vi "Module template.vi"(0 "Static input":T1(array[cluster])=[{"Times"=[], "Voltages"=[], "Enable Ch"=TRUE, "Hinge Points"=0}, {"Times"=[], "Voltages"=[], "Enable Ch"=TRUE, "Hinge Points"=0}, {"Times"=[], "Voltages"=[], "Enable Ch"=TRUE, "Hinge Points"=0}, {"Times"=[], "Voltages"=[], "Enable Ch"=TRUE, "Hinge Points"=0}, {"Times"=[], "Voltages"=[], "Enable Ch"=TRUE, "Hinge Points"=0}, {"Times"=[], "Voltages"=[], "Enable Ch"=TRUE, "Hinge Points"=0}, {"Times"=[], "Voltages"=[], "Enable Ch"=TRUE, "Hinge Points"=0}, {"Times"=[], "Voltages"=[], "Enable Ch"=TRUE, "Hinge Points"=0}, {"Times"=[], "Voltages"=[], "Enable Ch"=TRUE, "Hinge Points"=0}, {"Times"=[], "Voltages"=[], "Enable Ch"=TRUE, "Hinge Points"=0}, {"Times"=[], "Voltages"=[], "Enable Ch"=TRUE, "Hinge Points"=0}, {"Times"=[], "Voltages"=[], "Enable Ch"=TRUE, "Hinge Points"=0}, {"Times"=[], "Voltages"=[], "Enable Ch"=TRUE, "Hinge Points"=0}, {"Times"=[], "Voltages"=[], "Enable Ch"=TRUE, "Hinge Points"=0}, {"Times"=[], "Voltages"=[], "Enable Ch"=TRUE, "Hinge Points"=0}, {"Times"=[], "Voltages"=[], "Enable Ch"=TRUE, "Hinge Points"=0}, {"Times"=[], "Voltages"=[], "Enable Ch"=FALSE, "Hinge Points"=0}, {"Times"=[], "Voltages"=[], "Enable Ch"=FALSE, "Hinge Points"=0}, {"Times"=[], "Voltages"=[], "Enable Ch"=FALSE, "Hinge Points"=0}, {"Times"=[], "Voltages"=[], "Enable Ch"=FALSE, "Hinge Points"=0}, {"Times"=[], "Voltages"=[], "Enable Ch"=FALSE, "Hinge Points"=0}, {"Times"=[], "Voltages"=[], "Enable Ch"=FALSE, "Hinge Points"=0}, {"Times"=[], "Voltages"=[], "Enable Ch"=FALSE, "Hinge Points"=0}, {"Times"=[], "Voltages"=[], "Enable Ch"=TRUE, "Hinge Points"=0}] {"Voltages" format="%.2f"; "Times" format="%.2f"}, 1 "Absolute start time (ms)":dbl=1500.0 format="%.3f", 2 "GPIB Input":T3(array[cluster]) {"Module" items=["TTL high                                                                                 ", "TTL low                          ", "Camera Strobe                   ", "CMOT", "Defaults                           ", "Fluorescence pulse           ", "IP trap                         ", "Kinetics OD image          ", "Kinetics picture", "Kinetics probe pulse", "MOT light only                ", "MOT off                                   ", "MOT on                         ", "Move cart                      ", "OD image                     ", "Optical pumping          ", "Picture                             ", "Probe Pulse", "Quadrupole trap             ", "IP off", "Utility Module 02           ", "Utility Module 03           ", "Molasses          ", "Utility Module 04     ", "Utility Module 05     ", "Utility Module 06     ", "Utility Module 07     ", "Utility Module 08     ", "Utility Module 09     ", "Utility Module 10     ", "Static DAC", "GPIB"]; "Abs Start Time" format="%.3f"}, 3 "Read/Write":bool, 5 "Input":i64[][](array[numeric]), 7 "Static DAC Linear Ramps":T5(array[cluster]) {"DAC Channel" items=["0", "1", "2", "3", "4", "5", "6", "7", "8", "9", "10", "11", "12", "13", "14", "15", "16", "17", "18", "19", "20", "21", "22", "23"]}, 9 "Manual Array":T6(array[cluster])=[{"Time2 (ms)"="100", "Port2"=4, "Line2"=23, "Comments2"="", "Value2"=FALSE, "Enable2"=TRUE, "DAC value"="1"}, {"Time2 (ms)"="200", "Port2"=4, "Line2"=23, "Comments2"="", "Value2"=FALSE, "Enable2"=TRUE, "DAC value"="2"}] {"Line2" items=["0", "1", "2", "3", "4", "5", "6", "7", "8", "9", "10", "11", "12", "13", "14", "15", "16", "17", "18", "19", "20", "21", "22", "23", "24", "25", "26", "27", "28", "29", "30", "31"]; "Port2" items=["A", "B", "C", "D", "DAC", "GPIB"]}, 10 "Do Write/Read":bool, 12 "Do this?":bool=TRUE, 14 "filename":string="Utility Module 1") -> (4 "Static output":T1(array[cluster])=[{"Times"=[], "Voltages"=[], "Enable Ch"=TRUE, "Hinge Points"=0}, {"Times"=[], "Voltages"=[], "Enable Ch"=TRUE, "Hinge Points"=0}, {"Times"=[], "Voltages"=[], "Enable Ch"=TRUE, "Hinge Points"=0}, {"Times"=[], "Voltages"=[], "Enable Ch"=TRUE, "Hinge Points"=0}, {"Times"=[], "Voltages"=[], "Enable Ch"=TRUE, "Hinge Points"=0}, {"Times"=[], "Voltages"=[], "Enable Ch"=TRUE, "Hinge Points"=0}, {"Times"=[], "Voltages"=[], "Enable Ch"=TRUE, "Hinge Points"=0}, {"Times"=[], "Voltages"=[], "Enable Ch"=TRUE, "Hinge Points"=0}, {"Times"=[], "Voltages"=[], "Enable Ch"=TRUE, "Hinge Points"=0}, {"Times"=[], "Voltages"=[], "Enable Ch"=TRUE, "Hinge Points"=0}, {"Times"=[], "Voltages"=[], "Enable Ch"=TRUE, "Hinge Points"=0}, {"Times"=[], "Voltages"=[], "Enable Ch"=TRUE, "Hinge Points"=0}, {"Times"=[], "Voltages"=[], "Enable Ch"=TRUE, "Hinge Points"=0}, {"Times"=[], "Voltages"=[], "Enable Ch"=TRUE, "Hinge Points"=0}, {"Times"=[], "Voltages"=[], "Enable Ch"=TRUE, "Hinge Points"=0}, {"Times"=[], "Voltages"=[], "Enable Ch"=TRUE, "Hinge Points"=0}] {"Voltages" format="%.2f"; "Times" format="%.2f"}, 6 "Output":i64[][](array[numeric])=[[1700001, 3, 31, 0], [1700000, 3, 31, 1], [1600001, 3, 31, 0], [1600000, 3, 31, 1]], 13 "GPIB Output":T3(array[cluster]) {"Module" items=["TTL high                                                                                 ", "TTL low                          ", "Camera Strobe                   ", "CMOT", "Defaults                           ", "Fluorescence pulse           ", "IP trap                         ", "Kinetics OD image          ", "Kinetics picture", "Kinetics probe pulse", "MOT light only                ", "MOT off                                   ", "MOT on                         ", "Move cart                      ", "OD image                     ", "Optical pumping          ", "Picture                             ", "Probe Pulse", "Quadrupole trap             ", "IP off", "Utility Module 02           ", "Utility Module 03           ", "Molasses          ", "Utility Module 04     ", "Utility Module 05     ", "Utility Module 06     ", "Utility Module 07     ", "Utility Module 08     ", "Utility Module 09     ", "Utility Module 10     ", "Static DAC", "GPIB"]; "Abs Start Time" format="%.3f"}, 15 "Saved Cluster":T4={"Manual Array"=[{"Time2 (ms)"=100.0, "Port2"=4, "Line2"=23, "Comments2"="", "Value2"=FALSE, "Enable2"=TRUE, "DAC value"=1.0}, {"Time2 (ms)"=200.0, "Port2"=4, "Line2"=23, "Comments2"="", "Value2"=FALSE, "Enable2"=TRUE, "DAC value"=2.0}], "Static DAC Linear Ramps"=[]})   [LabVIEW 2017]
uses:
  globals/Modules global.vi
  globals/DIO board parameters global.vi
  globals/RIO and DAC defaults global.vi
panel:
  out "Static input 2":T1(array[cluster])
  out "Array":T2(array[cluster])=[{"Time2 (ms)"=100.0, "Port2"=4, "Line2"=23, "Comments2"="", "Value2"=FALSE, "Enable2"=TRUE, "DAC value"=1.0}, {"Time2 (ms)"=200.0, "Port2"=4, "Line2"=23, "Comments2"="", "Value2"=FALSE, "Enable2"=TRUE, "DAC value"=2.0}]
  out "Path":path=path "E:/Debbie/experiment stuff/B231/24 Experiment Control/modules and sub-vi's/quad trap"
  out "appended path":path=path "E:/Debbie/experiment stuff/B231/24 Experiment Control/modules and sub-vi's/backups/Helmholtz1 28_Apr_2006"
  out "Comments":string[](array[string])
  out "Value":bool[](array[boolean])
  out "Line":i32[](array[numeric])
  out "Port":i32[](array[numeric])
  out "Time":dbl[](array[numeric]) format="%.3f"
  # "manual button (not connected on icon)\nIf you set this to True, be sure to set it back to False afterward."
  # "Time                   Port        Line       Value  Enable  DAC voltage  Comments"
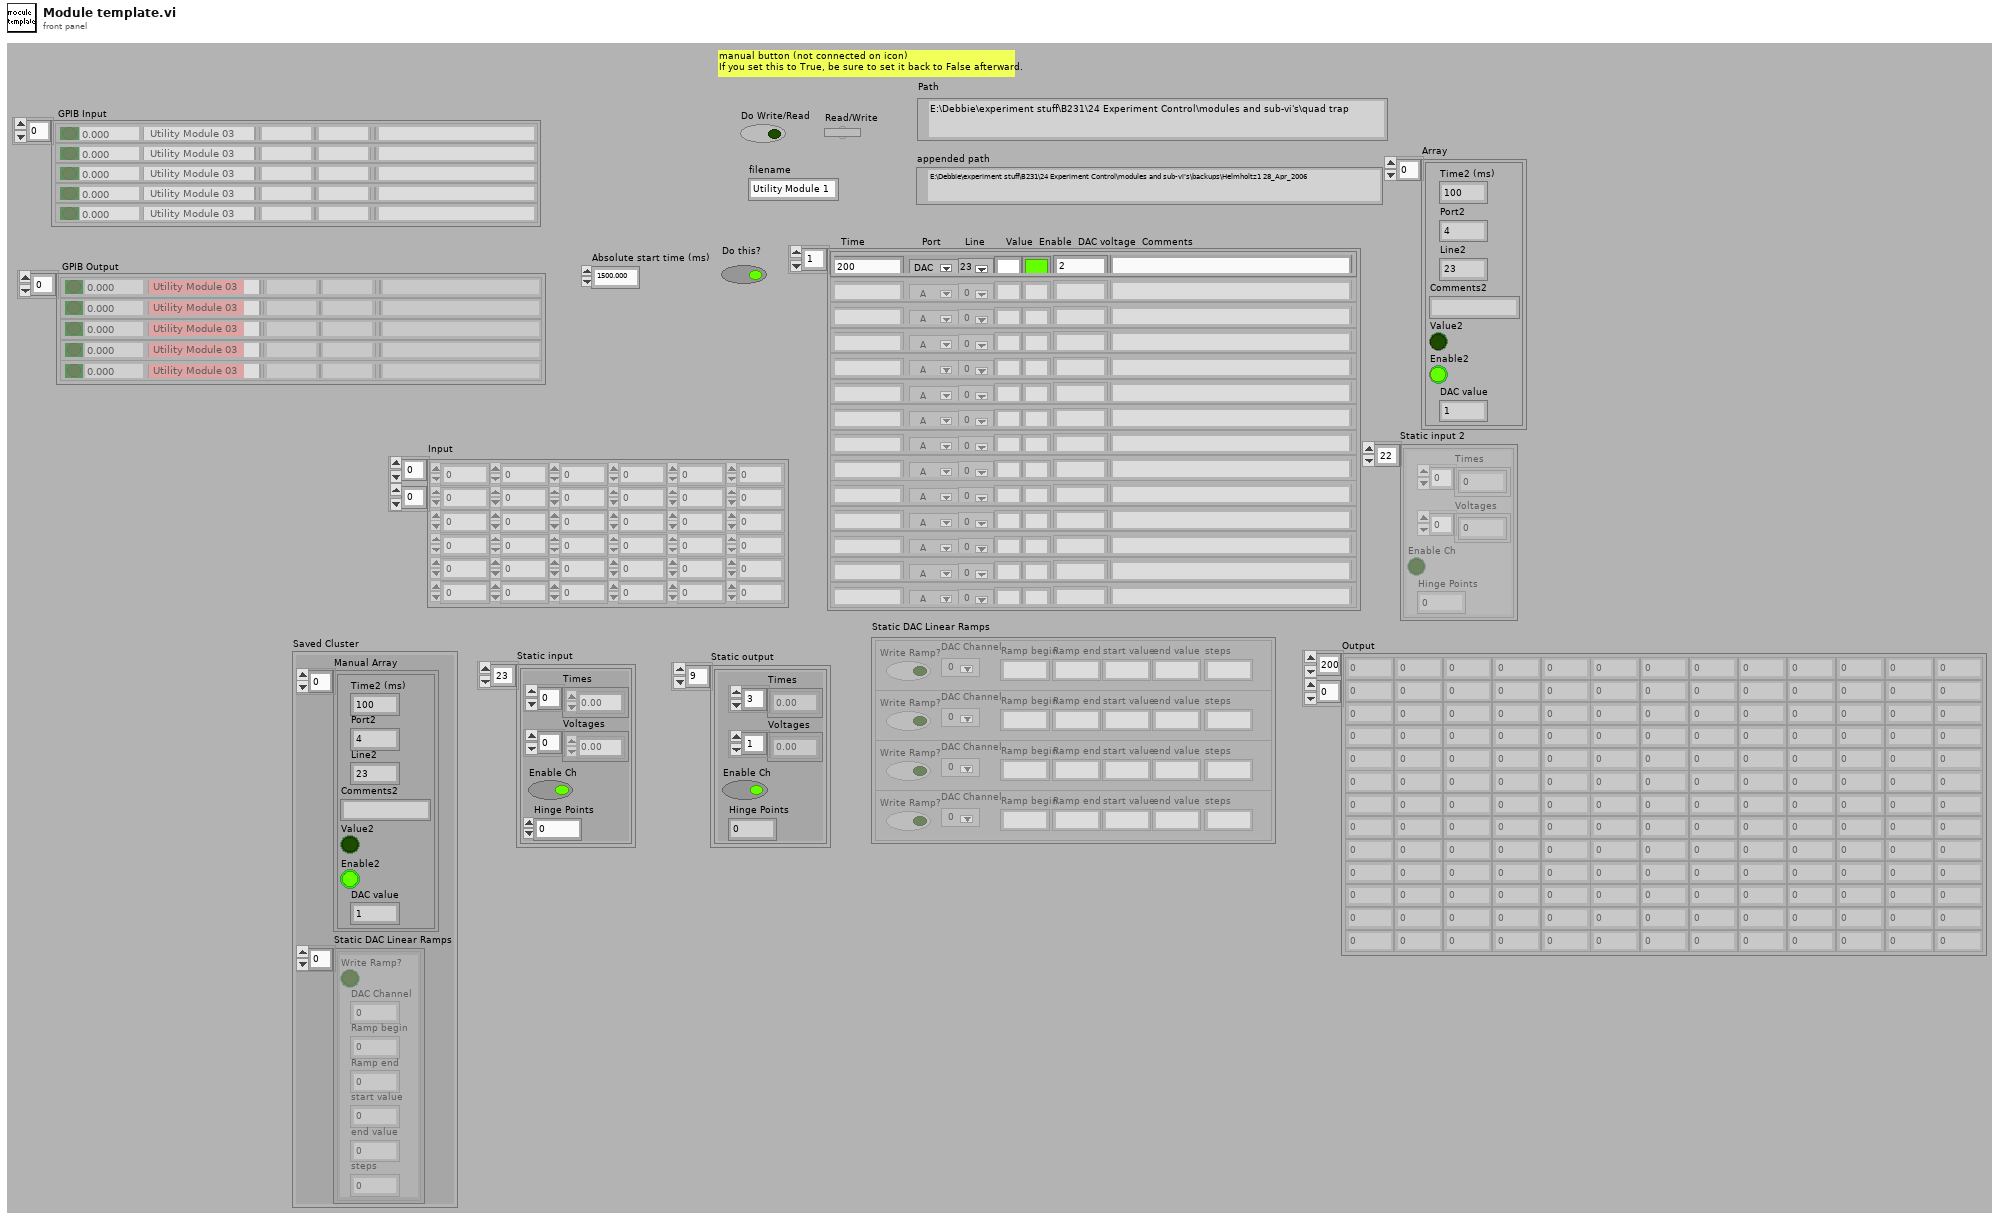
[diagram p1: front panel]
types:
  T1 = cluster{"Times":dbl[], "Voltages":dbl[], "Enable Ch":bool, "Hinge Points":u8}[]
  T2 = cluster{"Time2 (ms)":dbl, "Port2":u16, "Line2":u16, "Comments2":string, "Value2":bool, "Enable2":bool, "DAC value":dbl}[]
  T3 = cluster{"Enable":bool, "Abs Start Time":dbl, "Module":u16, "String":string, "Array":string[]}[]
  T4 = cluster{"Manual Array":cluster{"Time2 (ms)":dbl, "Port2":u16, "Line2":u16, "Comments2":string, "Value2":bool, "Enable2":bool, "DAC value":dbl}[], "Static DAC Linear Ramps":cluster{"Write Ramp?":bool, "DAC Channel":i16, "Ramp begin":dbl, "Ramp end":dbl, "start value":dbl, "end value":dbl, "steps":i16}[]}
  T5 = cluster{"Write Ramp?":bool, "DAC Channel":i16, "Ramp begin":string, "Ramp end":string, "start value":string, "end value":string, "steps":string}[]
  T6 = cluster{"Time2 (ms)":string, "Port2":u16, "Line2":u16, "Comments2":string, "Value2":bool, "Enable2":bool, "DAC value":string}[]
  T7 = cluster{"Write Ramp?":bool, "DAC Channel":i16, "Ramp begin":dbl, "Ramp end":dbl, "start value":dbl, "end value":dbl, "steps":i16}[]
  T8 = cluster{"Write Ramp?":bool, "DAC Channel":i16, "Ramp begin":dbl, "Ramp end":dbl, "start value":dbl, "end value":dbl, "steps":i16}
  T9 = cluster{"Time2 (ms)":dbl, "Port2":u16, "Line2":u16, "Comments2":string, "Value2":bool, "Enable2":bool, "DAC value":dbl}
  T10 = cluster{cluster{"Time2 (ms)":dbl, "Port2":u16, "Line2":u16, "Comments2":string, "Value2":bool, "Enable2":bool, "DAC value":dbl}[], cluster{"Write Ramp?":bool, "DAC Channel":i16, "Ramp begin":dbl, "Ramp end":dbl, "start value":dbl, "end value":dbl, "steps":i16}[]}
  T11 = enum32{"existing file", "new file", "new or existing file", "existing dir", "new dir", "new or existing dir", "existing file (use LLBs)", "new file (use LLBs)", "new or existing file (use LLBs)", "new or existing file or directory (use LLBs)"}
  T12 = enum16{"open", "replace", "create", "open or create", "replace or create", "replace or create with confirmation"}
  T13 = cluster{"Time2 (ms)":string, "Port2":u16, "Line2":u16, "Comments2":string, "Value2":bool, "Enable2":bool, "DAC value":string}
  T14 = cluster{"Write Ramp?":bool, "DAC Channel":i16, "Ramp begin":string, "Ramp end":string, "start value":string, "end value":string, "steps":string}
  T15 = cluster{"Enable":bool, "Abs Start Time":dbl, "Module":u16, "String":string, "Array":string[]}
  T16 = cluster{"Times":dbl[], "Voltages":dbl[], "Enable Ch":bool, "Hinge Points":u8}
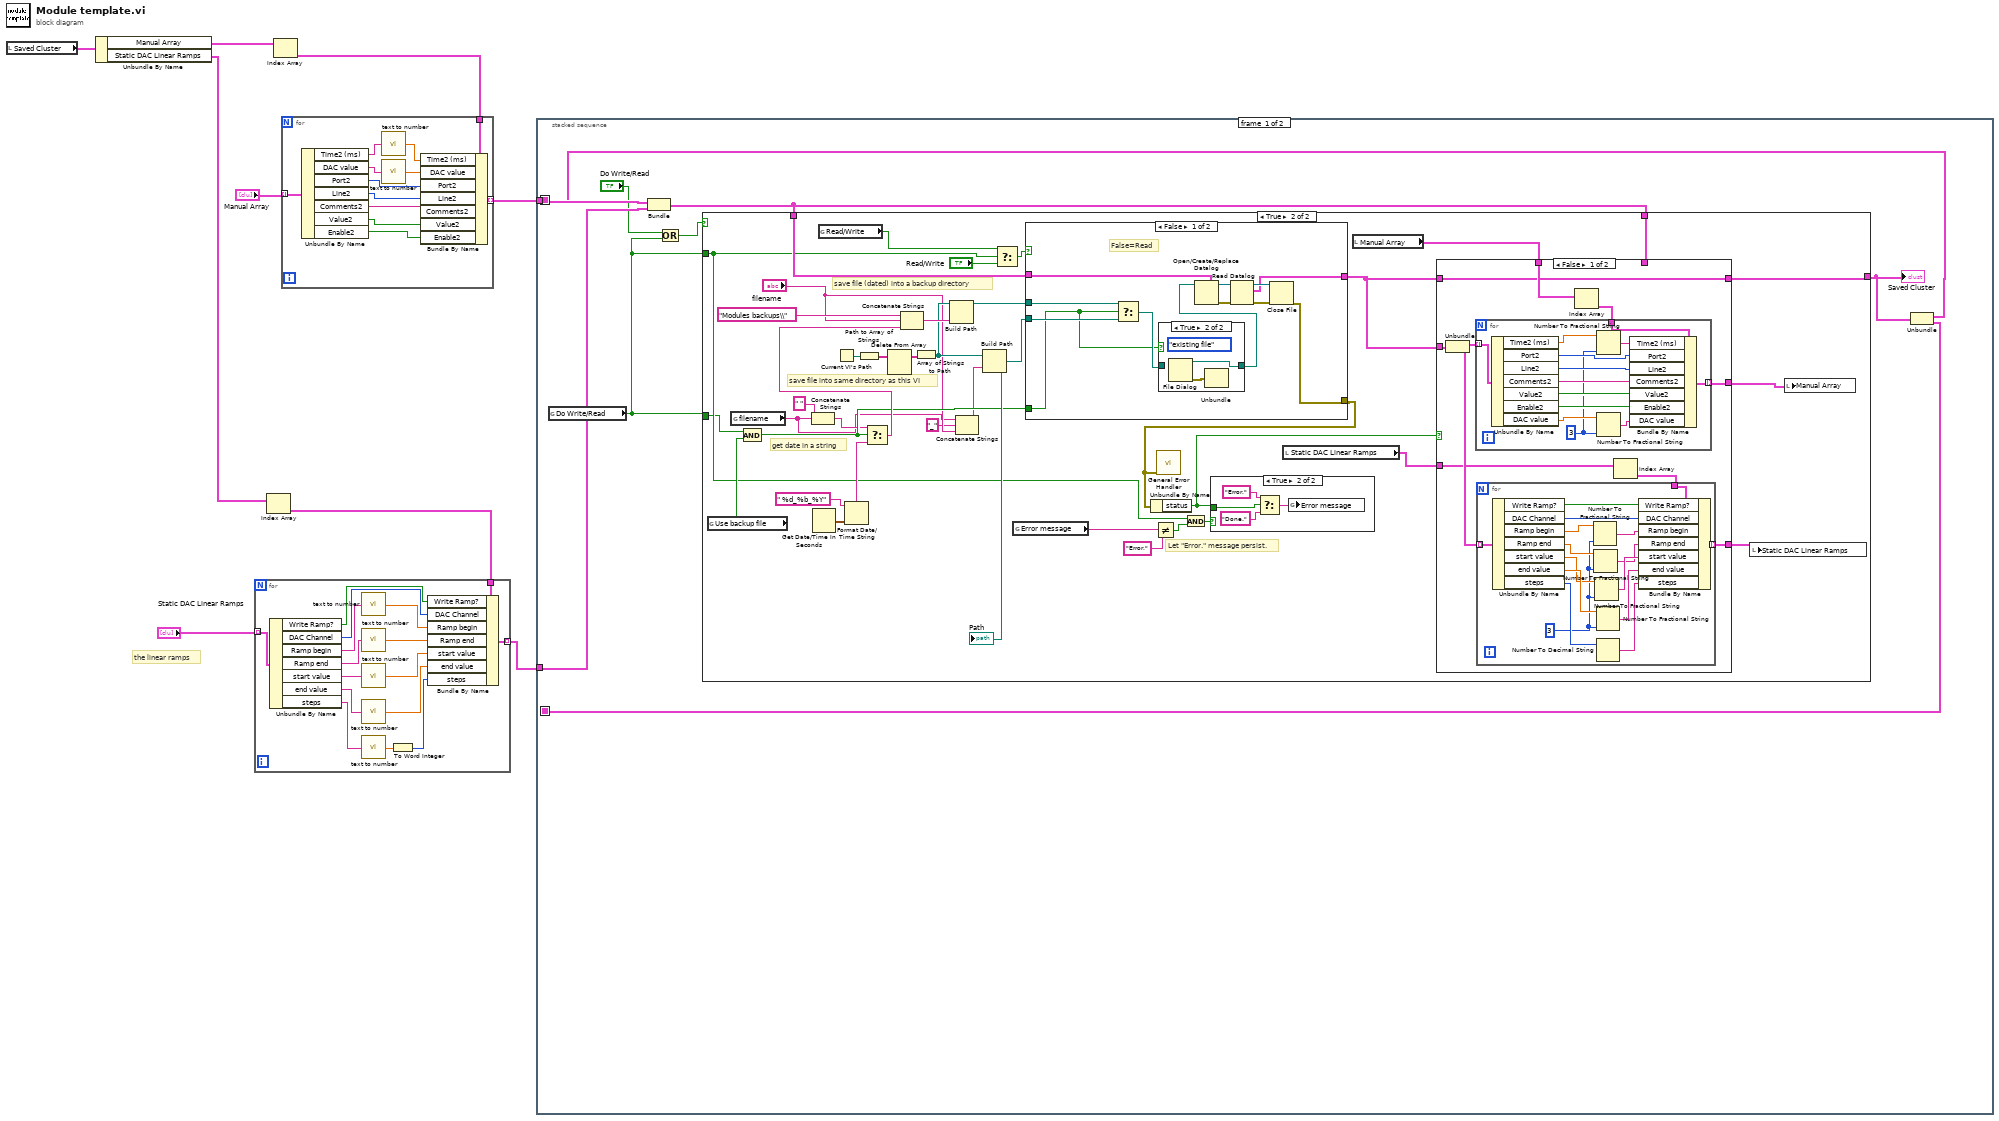
[diagram p0: block diagram]
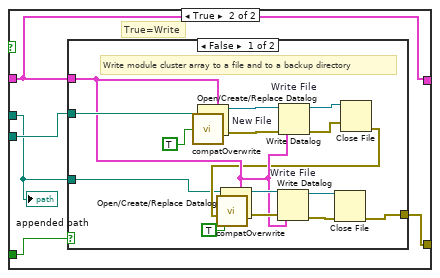
[diagram p6: hidden frame]
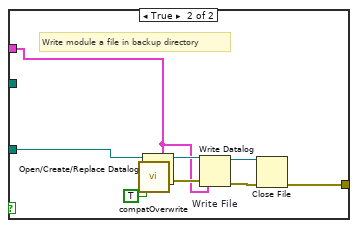
[diagram p7: hidden frame]
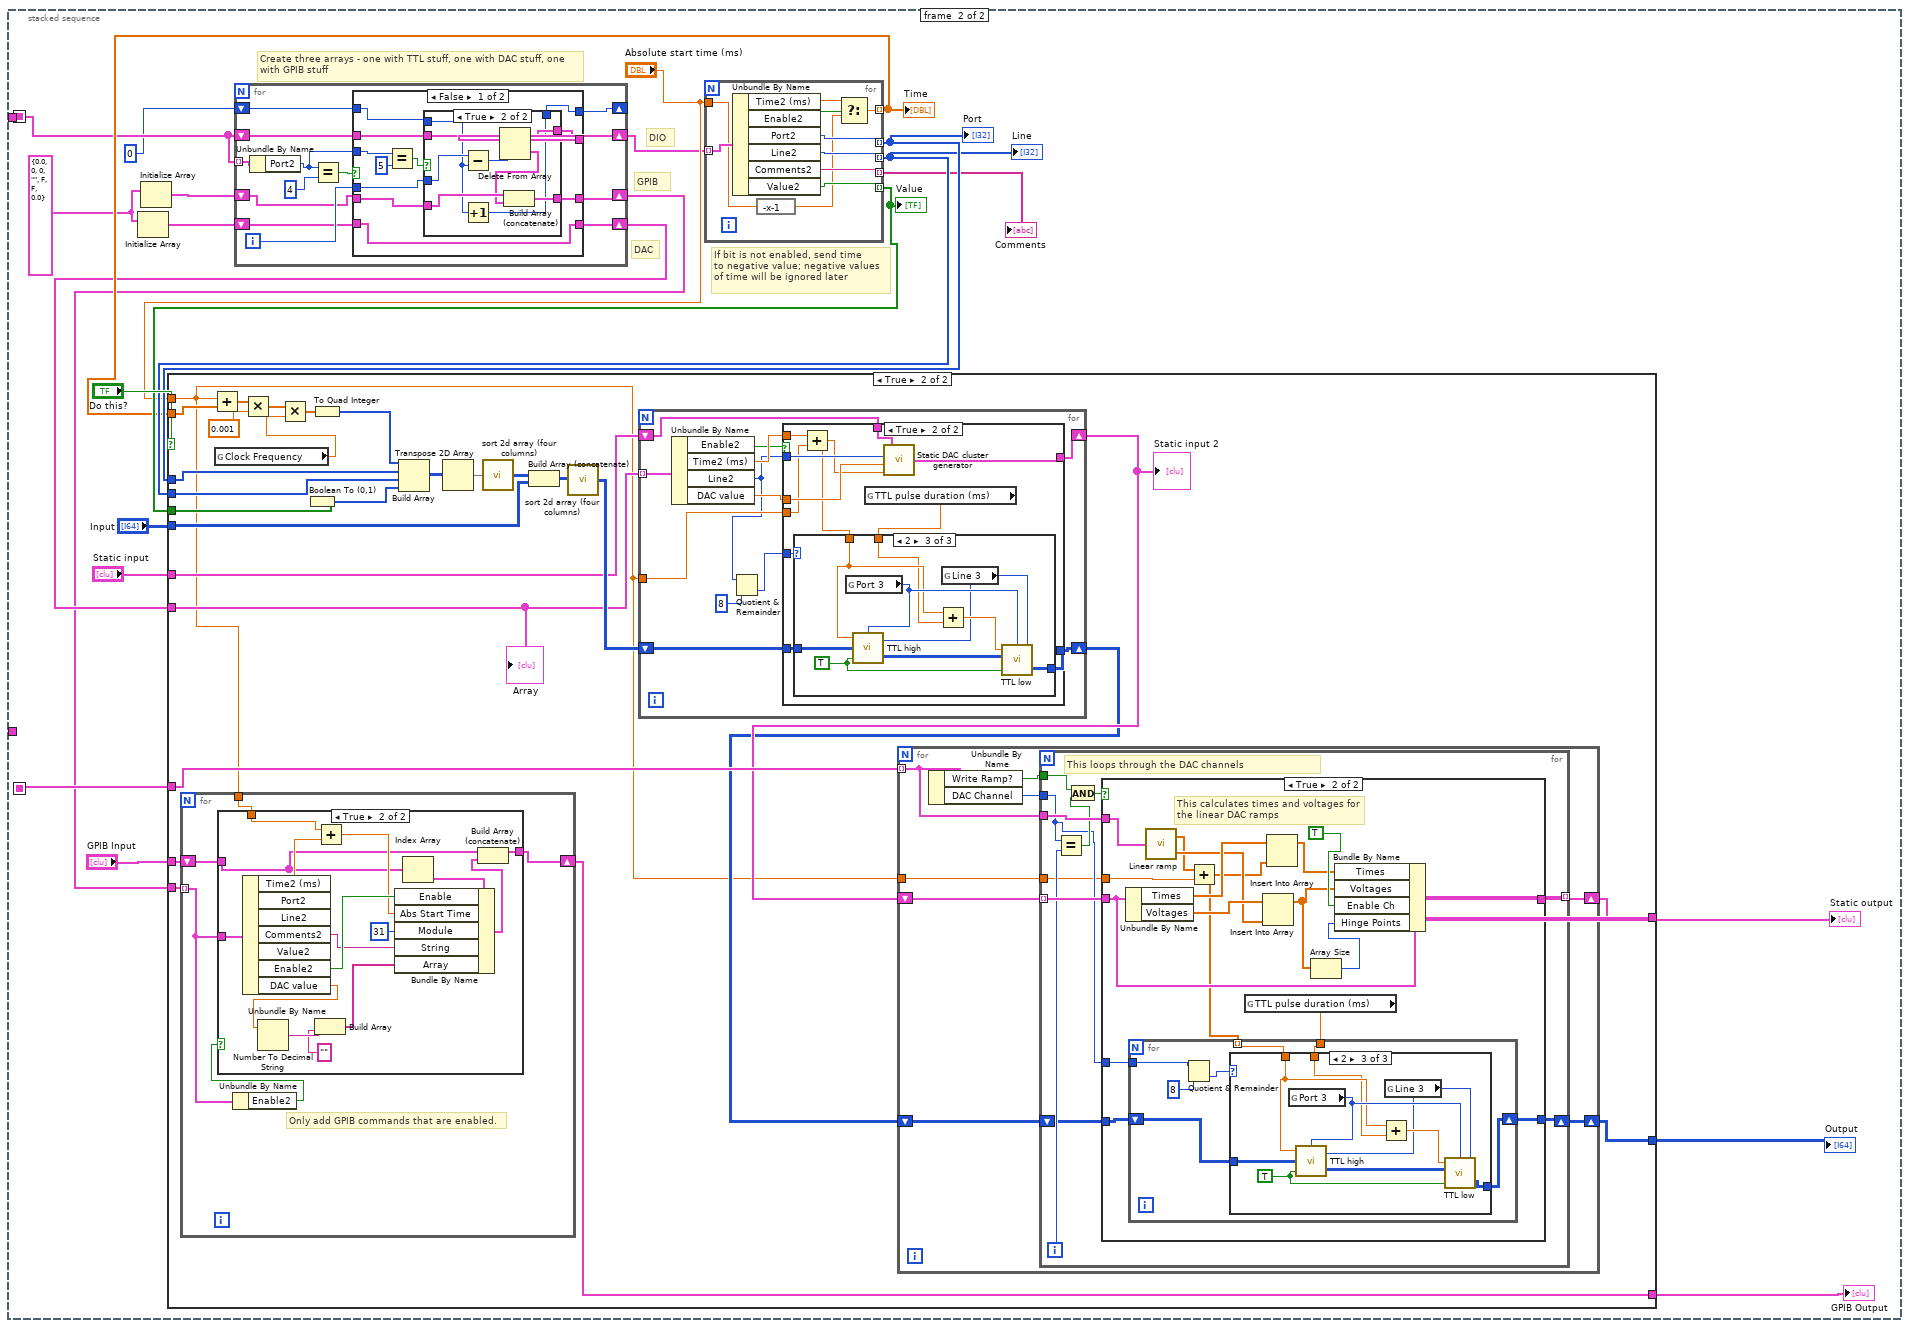
[diagram p8: hidden frame]
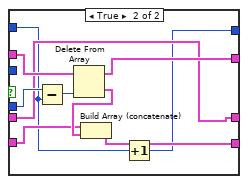
[diagram p10: hidden frame]
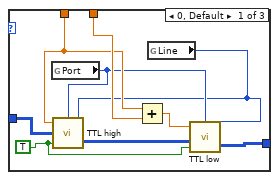
[diagram p14: hidden frame]
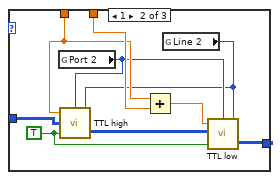
[diagram p15: hidden frame]
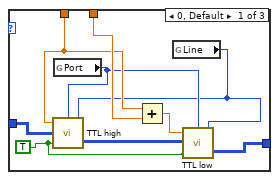
[diagram p17: hidden frame]
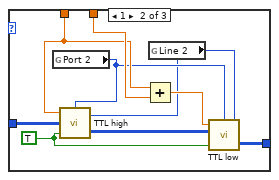
[diagram p18: hidden frame]
diagram:
  # "the linear ramps"
  n1 = local read "Saved Cluster"() -> (w5:T4)
  n2 = Unbundle By Name(w5) -> ("Manual Array"=w3:T2, "Static DAC Linear Ramps"=w1:T7)
  n3 = Index Array(array=w1) -> (element=w2:T8)  [unwired: 1 in]
  n4 = for {
    tunnel: "Static DAC Linear Ramps" -> [w25] mode=indexing
    tunnel: [w24] -> w6 mode=indexing
    tunnel: w2 -> [w10]
    n5 = Unbundle By Name(w25) -> ("Write Ramp?"=w23:bool, "DAC Channel"=w22:i16, "Ramp begin"=w21:string, "Ramp end"=w20:string, "start value"=w19:string, "end value"=w18:string, "steps"=w17:string)
    n6 = call "text to number.vi"("text"=w21) -> ("number"=w16:dbl)
    n7 = call "text to number.vi"("text"=w20) -> ("number"=w15:dbl)
    n8 = call "text to number.vi"("text"=w19) -> ("number"=w14:dbl)
    n9 = call "text to number.vi"("text"=w18) -> ("number"=w13:dbl)
    n10 = call "text to number.vi"("text"=w17) -> ("number"=w12:dbl)
    n11 = To Word Integer(number=w12) -> (16bit integer=w11:i16)
    n12 = Bundle By Name(cluster=w10, "Write Ramp?"=w23, "DAC Channel"=w22, "Ramp begin"=w16, "Ramp end"=w15, "start value"=w14, "end value"=w13, "steps"=w11) -> (w24:T8)
  }
  n13 = Index Array(array=w3) -> (element=w4:T9)  [unwired: 1 in]
  n14 = for {
    tunnel: "Manual Array" -> [w37] mode=indexing
    tunnel: [w27] -> w8 mode=indexing
    tunnel: w4 -> [w26]
    n15 = Unbundle By Name(w37) -> ("Time2 (ms)"=w31:string, "DAC value"=w29:string, "Port2"=w32:u16, "Line2"=w33:u16, "Comments2"=w34:string, "Value2"=w36:bool, "Enable2"=w35:bool)
    n16 = call "text to number.vi"("text"=w31) -> ("number"=w30:dbl)
    n17 = call "text to number.vi"("text"=w29) -> ("number"=w28:dbl)
    n18 = Bundle By Name(cluster=w26, "Time2 (ms)"=w30, "DAC value"=w28, "Port2"=w32, "Line2"=w33, "Comments2"=w34, "Value2"=w36, "Enable2"=w35) -> (w27:T9)
  }
  n19 = stacked-sequence {
    seq-local: [w43 _] -> [_ w188]
    seq-local: [w39 _] -> [_ w190]
    tunnel: w8 -> [w46 _]
    tunnel: w6 -> [w45 _]
    frame #0 {
      n20 = global read "Modules global.vi" "Do Write/Read"() -> (w40:bool)
      n21 = Bundle(w46, w45) -> (w38:T10)  [unwired: 1 in]
      n22 = Or(x="Do Write/Read", y=w40) -> (x .or. y?=w42:bool)
      n23 = case shown="True" w42 {
        tunnel: w38 -> [w47 w78]
        tunnel: [w47 w50] -> w44
        tunnel: w40 -> [_ w62]
        tunnel: w40 -> [_ w61]
        tunnel: w38 -> [_ w49]
        frame False {
        }
        frame True {
          # "Let \"Error.\" message persist."
          # "get date in a string"
          # "save file (dated) into a backup directory"
          # "save file into same directory as this VI"
          n24 = global read "Modules global.vi" "Use backup file"() -> (w75:bool)
          n25 = global read "Modules global.vi" "filename"() -> (w54:string)
          n26 = Compound Arithmetic op=AND(w61, w75) -> (w69:bool)
          n27 = Concatenate Strings(" " ("string"), w54) -> (w67:string)
          n28 = Get Date/Time In Seconds() -> (seconds since 1Jan1904=w72:timestamp)
          n29 = global read "Modules global.vi" "Read/Write"() -> (w74:bool)
          n30 = Current VI's Path() -> (path=w79:path)
          n31 = Format Date/Time String(time format string (%c)=" %d_%b_%Y", seconds (now)=w72) -> (date/time string=w71:string)  [unwired: 1 in]
          n32 = Path to Array of Strings(0:w79) -> (2:w80:string[])  [unwired: 1 out]
          n33 = Select(t=w67, s=w69, f=w71) -> (s? t:f=w70:string)
          n34 = Delete From Array(array=w80) -> (array with subset deleted=w81:string[])  [unwired: 2 in, 1 out]
          n35 = Concatenate Strings("Modules backups\\" ("Substring"), "filename", w70) -> (w84:string)
          n36 = Array of Strings to Path(0:w81) -> (2:w83:path)  [unwired: 1 in]
          n37 = Build Path(base path=w83, name or relative path=w84) -> (appended path=w86:path)
          n38 = Concatenate Strings(w54, "_" ("string"), "filename") -> (w53:string)
          n39 = Build Path(base path=w83, name or relative path=w53) -> (appended path=w85:path)
          "Path" <- w85
          n40 = Select(t=w74, s=w62, f="Read/Write") -> (s? t:f=w76:bool)
          n41 = global read "Modules global.vi" "Error message"() -> (w66:string)
          n42 = case shown="False" w76 {
            tunnel: [w144 w152] -> w48
            tunnel: w85 -> [w137 w151]
            tunnel: w86 -> [w136 w149]
            tunnel: w78 -> [w140 w150]
            tunnel: [w138 w150] -> w51
            tunnel: w69 -> [w133 w148]
            frame False {
              # "False=Read"
              n43 = Select(t=w136, s=w133, f=w137) -> (s? t:f=w135:path)
              n44 = case shown="True" w133 {
                tunnel: w135 -> [w145 _]
                tunnel: [w145 w147] -> w134
                frame False {
                }
                frame True {
                  (unwired) T11."existing file" ("select mode (2)")
                  n45 = File Dialog() -> (0:w146:errorcluster, 3:w147:path)  [unwired: 7 in, 2 out]
                  n46 = Unbundle(w146) -> ()  [unwired: 3 out]
                }
              }
              n47 = Open/Create/Replace Datalog(5:w140, 11:w134) -> (0:w142:errorcluster, 3:w139:refnum<k1>)  [unwired: 4 in, 1 out]
              n48 = Read Datalog(4:w142, 7:w139) -> (0:w143:errorcluster, 2:w138:T10, 3:w141:refnum<k1>)  [unwired: 1 in]
              n49 = Close File(refnum=w141, error in=w143) -> (error out=w144:errorcluster)  [unwired: 1 out]
            }
            frame True {
              # "True=Write"
              n50 = case shown="False" w148 {
                tunnel: [w162 w173] -> w152
                tunnel: w151 -> [w160 _]
                tunnel: w150 -> [w158 w171]
                tunnel: w149 -> [w155 w172]
                frame False {
                  # "Write module cluster array to a file and to a backup directory"
                  n51 = call <vilib>:"compatOverwrite.vi"("overwrite (F)"=TRUE) -> ("overwrite?"=w153:T12)
                  n52 = Open/Create/Replace Datalog "New File"(5:w158, 10:w153, 11:w160) -> (0:w165:errorcluster, 3:w159:refnum<k1>)  [unwired: 3 in, 1 out]
                  n53 = call <vilib>:"compatOverwrite.vi"("overwrite (F)"=TRUE) -> ("overwrite?"=w154:T12)
                  n54 = Write Datalog "Write File"(4:w165, 6:w158, 7:w159) -> (0:w166:errorcluster, 3:w168:refnum<k1>)
                  n55 = Close File(refnum=w168, error in=w166) -> (error out=w157:errorcluster)  [unwired: 1 out]
                  n56 = Open/Create/Replace Datalog ("New File")(5:w158, 8:w157, 10:w154, 11:w155) -> (0:w163:errorcluster, 3:w161:refnum<k1>)  [unwired: 2 in, 1 out]
                  n57 = Write Datalog "Write File"(4:w163, 6:w158, 7:w161) -> (0:w164:errorcluster, 3:w167:refnum<k1>)
                  n58 = Close File(refnum=w167, error in=w164) -> (error out=w162:errorcluster)  [unwired: 1 out]
                }
                frame True {
                  # "Write module a file in backup directory"
                  n59 = call <vilib>:"compatOverwrite.vi"("overwrite (F)"=TRUE) -> ("overwrite?"=w170:T12)
                  n60 = Open/Create/Replace Datalog ("New File")(5:w171, 10:w170, 11:w172) -> (0:w176:errorcluster, 3:w175:refnum<k1>)  [unwired: 3 in, 1 out]
                  n61 = Write Datalog "Write File"(4:w176, 6:w171, 7:w175) -> (0:w177:errorcluster, 3:w178:refnum<k1>)
                  n62 = Close File(refnum=w178, error in=w177) -> (error out=w173:errorcluster)  [unwired: 1 out]
                }
              }
              "appended path" <- w149
            }
          }
          n63 = Unbundle By Name(w48) -> ("status"=w52:bool)
          n64 = Not Equal?(x=w66, y="Error." ("Error message")) -> (x != y?=w63:bool)
          n65 = call <vilib>:"General Error Handler.vi"("error in (no error)"=w48) -> ()  [unwired: 10 in, 5 out]
          n66 = And(x=w62, y=w63) -> (x .and. y?=w64:bool)
          n67 = case shown="True" w64 {
            tunnel: w52 -> [_ w131]
            frame False {
            }
            frame True {
              n68 = Select(t="Error." ("Error message"), s=w131, f="Done." ("Error message")) -> (s? t:f=w132:string)
              n69 = global write "Modules global.vi" "Error message"(w132) -> ()
            }
          }
          n70 = local read "Static DAC Linear Ramps"() -> (w58:T5)
          n71 = local read "Manual Array"() -> (w60:T6)
          n72 = case shown="False" w52 {
            tunnel: w51 -> [w96 _]
            tunnel: w60 -> [w93 w128]
            tunnel: [w91 w128] -> w59
            tunnel: w58 -> [w90 w127]
            tunnel: [w88 w127] -> w57
            tunnel: w51 -> [w87 _]
            tunnel: [w87 w126] -> w50
            tunnel: w49 -> [_ w126]
            frame False {
              n73 = Unbundle(w96) -> (w95:T2, w94:T7)
              n74 = Index Array(array=w93) -> (element=w92:T13)  [unwired: 1 in]
              n75 = for {
                tunnel: w95 -> [w125] mode=indexing
                tunnel: w92 -> [w124]
                tunnel: [w114] -> w91 mode=indexing
                w113 = i16 3 ("precision (6)")
                n76 = Unbundle By Name(w125) -> ("Time2 (ms)"=w117:dbl, "Port2"=w122:u16, "Line2"=w121:u16, "Comments2"=w120:string, "Value2"=w119:bool, "Enable2"=w118:bool, "DAC value"=w116:dbl)
                n77 = Number To Fractional String(number=w117, precision (6)=w113) -> (F-format string=w123:string)  [unwired: 2 in]
                n78 = Number To Fractional String(number=w116, precision (6)=w113) -> (F-format string=w115:string)  [unwired: 2 in]
                n79 = Bundle By Name(cluster=w124, "Time2 (ms)"=w123, "Port2"=w122, "Line2"=w121, "Comments2"=w120, "Value2"=w119, "Enable2"=w118, "DAC value"=w115) -> (w114:T13)
              }
              n80 = Index Array(array=w90) -> (element=w89:T14)  [unwired: 1 in]
              n81 = for {
                tunnel: w94 -> [w112] mode=indexing
                tunnel: w89 -> [w111]
                tunnel: [w98] -> w88 mode=indexing
                w97 = i16 3 ("precision (6)")
                n82 = Unbundle By Name(w112) -> ("Write Ramp?"=w110:bool, "DAC Channel"=w109:i16, "Ramp begin"=w99:dbl, "Ramp end"=w102:dbl, "start value"=w104:dbl, "end value"=w106:dbl, "steps"=w108:i16)
                n83 = Number To Fractional String(number=w99, precision (6)=w97) -> (F-format string=w100:string)  [unwired: 2 in]
                n84 = Number To Fractional String(number=w102, precision (6)=w97) -> (F-format string=w101:string)  [unwired: 2 in]
                n85 = Number To Fractional String(number=w104, precision (6)=w97) -> (F-format string=w103:string)  [unwired: 2 in]
                n86 = Number To Fractional String(number=w106, precision (6)=w97) -> (F-format string=w105:string)  [unwired: 2 in]
                n87 = Number To Decimal String(number=w108) -> (decimal integer string=w107:string)  [unwired: 1 in]
                n88 = Bundle By Name(cluster=w111, "Write Ramp?"=w110, "DAC Channel"=w109, "Ramp begin"=w100, "Ramp end"=w101, "start value"=w103, "end value"=w105, "steps"=w107) -> (w98:T14)
              }
            }
            frame True {
            }
          }
          n89 = local write "Static DAC Linear Ramps"(w57) -> ()
          n90 = local write "Manual Array"(w59) -> ()
        }
      }
      "Saved Cluster" <- w44
      n91 = Unbundle(w44) -> (w39:T2, w43:T7)
    }
    frame #1 {
      w183 = T9 {"Time2 (ms)"=0.0, "Port2"=0, "Line2"=0, "Comments2"="", "Value2"=FALSE, "Enable2"=FALSE, "DAC value"=0.0} ("manual cluster")
      # "GPIB"
      # "DAC"
      # "DIO"
      # "Create three arrays - one with TTL stuff, one with DAC stuff, one with GPIB stuff"
      # "If bit is not enabled, send time\nto negative value; negative values\nof time will be ignored later"
      n92 = Initialize Array(w183) -> (w192:T2)  [unwired: 1 in]
      n93 = Initialize Array(w183) -> (w182:T2)  [unwired: 1 in]
      n94 = for {
        tunnel: w190 -> [w207] mode=indexing
        shift-right: [w212] -> w191
        shift-left: w190 -> [w213]
        shift-right: [w205] -> w189
        shift-left: w192 -> [w208]
        shift-right: [w203] -> w181
        shift-left: w182 -> [w204]
        shift-right: [w201] -> _
        shift-left: u16 0 ("y") -> [w202]
        i -> [w209]
        n95 = Unbundle By Name(w207) -> ("Port2"=w206:u16)
        n96 = Equal?(x=w206, y=u16 4) -> (x = y?=w211:bool)
        n97 = case shown="False" w211 {
          tunnel: w213 -> [w222 w246]
          tunnel: [w221 w245] -> w212
          tunnel: w209 -> [w219 w242]
          tunnel: [w217 w243] -> w205
          tunnel: w208 -> [w217 w239]
          tunnel: w206 -> [w223 _]
          tunnel: w204 -> [w218 w240]
          tunnel: [w216 w240] -> w203
          tunnel: w202 -> [w215 w238]
          tunnel: [w214 w237] -> w201
          frame False {
            n98 = Equal?(x=w223, y=u16 5) -> (x = y?=w220:bool)
            n99 = case shown="True" w220 {
              tunnel: w222 -> [w227 w235]
              tunnel: w218 -> [w226 w232]
              tunnel: [w227 w234] -> w221
              tunnel: [w226 w233] -> w216
              tunnel: w219 -> [_ w236]
              tunnel: w215 -> [w225 w229]
              tunnel: [w225 w228] -> w214
              frame False {
              }
              frame True {
                n100 = Subtract(x=w236, y=w229) -> (x-y=w230:i32)
                n101 = Increment(x=w229) -> (x+1=w228:u16)
                n102 = Delete From Array(array=w235, index=w230) -> (deleted portion=w231:T9, array with subset deleted=w234:T2)  [unwired: 1 in]
                n103 = Build Array (concatenate)(w232, w231) -> (w233:T2)
              }
            }
          }
          frame True {
            n104 = Subtract(x=w242, y=w238) -> (x-y=w241:i32)
            n105 = Delete From Array(array=w246, index=w241) -> (deleted portion=w244:T9, array with subset deleted=w245:T2)  [unwired: 1 in]
            n106 = Build Array (concatenate)(w239, w244) -> (w243:T2)
            n107 = Increment(x=w238) -> (x+1=w237:u16)
          }
        }
      }
      n108 = for {
        tunnel: w191 -> [w256] mode=indexing
        tunnel: [w251] -> w195 mode=indexing
        tunnel: [w255] -> w199 mode=indexing
        tunnel: [w254] -> w198 mode=indexing
        tunnel: [w253] -> w197 mode=indexing
        tunnel: [w252] -> w196 mode=indexing
        tunnel: "Absolute start time (ms)" -> [w247]
        n109 = Unbundle By Name(w256) -> ("Time2 (ms)"=w250:dbl, "Enable2"=w248:bool, "Port2"=w255:u16, "Line2"=w254:u16, "Comments2"=w253:string, "Value2"=w252:bool)
        n110 = expression code="-x-1"(w247) -> (w249:dbl)
        n111 = Select(t=w250, s=w248, f=w249) -> (s? t:f=w251:dbl)
      }
      "Time" <- w195
      "Port" <- w199
      "Line" <- w198
      "Comments" <- w197
      "Value" <- w196
      n112 = case shown="True" "Do this?" {
        tunnel: w195 -> [_ w285]
        tunnel: w199 -> [_ w278]
        tunnel: w198 -> [_ w277]
        tunnel: w196 -> [_ w284]
        tunnel: "Static input" -> [w259 w272]
        tunnel: w189 -> [_ w271]
        tunnel: "Absolute start time (ms)" -> [_ w261]
        tunnel: w188 -> [_ w270]
        tunnel: [w259 w268] -> w187
        tunnel: [w258 w265] -> w185
        tunnel: "Input" -> [w258 w267]
        tunnel: "GPIB Input" -> [w257 w263]
        tunnel: w181 -> [_ w264]
        tunnel: [w257 w262] -> w180
        frame False {
        }
        frame True {
          n113 = for {
            tunnel: w264 -> [w289] mode=indexing
            shift-right: [w291] -> w262
            shift-left: w263 -> [w292]
            tunnel: w261 -> [w290]
            # "Only add GPIB commands that are enabled."
            n114 = Unbundle By Name(w289) -> ("Enable2"=w288:bool)
            n115 = case shown="True" w288 {
              tunnel: w292 -> [w293 w294]
              tunnel: [w293 w299] -> w291
              tunnel: w290 -> [_ w298]
              tunnel: w289 -> [_ w295]
              frame False {
              }
              frame True {
                n116 = Unbundle By Name(w295) -> ("Time2 (ms)"=w296:dbl, "Comments2"=w305:string, "Enable2"=w307:bool, "DAC value"=w301:dbl)  [unwired: 3 out]
                n117 = Number To Decimal String(number=w301) -> (decimal integer string=w304:string)  [unwired: 1 in]
                n118 = Build Array(w304, "" ("element")) -> (w302:string[])
                n119 = Add(x=w298, y=w296) -> (x+y=w297:dbl)
                n120 = Index Array(array=w294) -> (element=w308:T15)  [unwired: 1 in]
                n121 = Bundle By Name(cluster=w308, "Enable"=w307, "Abs Start Time"=w297, "Module"=u16 31, "String"=w305, "Array"=w302) -> (w300:T15)
                n122 = Build Array (concatenate)(w294, w300) -> (w299:T3)
              }
            }
          }
          n123 = Add(x=w261, y=w285) -> (x+y=w282:dbl[])
          n124 = global read "DIO board parameters global.vi" "Clock Frequency"() -> (w260:dbl)
          n125 = Multiply(x=w282, y=0.001) -> (x*y=w286:dbl[])
          n126 = Multiply(x=w286, y=w260) -> (x*y=w283:dbl[])
          n127 = Boolean To (0,1)(Boolean=w284) -> (0, 1=w276:i16[])
          n128 = To Quad Integer(1:w283) -> (0:w279:i64[])
          n129 = Build Array(w279, w278, w277, w276) -> (w281:i64[][])
          n130 = Transpose 2D Array(2D array=w281) -> (transposed array=w280:i64[][])
          n131 = call "sort 2d array (four columns).vi"("2D array to sort"=w280) -> ("Sorted array"=w275:i64[][])
          n132 = Build Array (concatenate)(w275, w267) -> (w274:i64[][])
          n133 = call "sort 2d array (four columns).vi"("2D array to sort"=w274) -> ("Sorted array"=w273:i64[][])
          n134 = for {
            shift-right: [w388] -> w269
            shift-left: w272 -> [w390]
            tunnel: w271 -> [w391] mode=indexing
            shift-right: [w387] -> w266
            shift-left: w273 -> [w392]
            tunnel: w261 -> [w386]
            n135 = Unbundle By Name(w391) -> ("Enable2"=w384:bool, "Time2 (ms)"=w385:dbl, "Line2"=w383:u16, "DAC value"=w389:dbl)
            n136 = Quotient & Remainder(x=w383, y=8) -> (floor(x/y)=w381:i32)  [unwired: 1 out]
            n137 = case shown="True" w384 {
              tunnel: w392 -> [w393 w405]
              tunnel: w390 -> [w394 w404]
              tunnel: w389 -> [_ w403]
              tunnel: w383 -> [_ w402]
              tunnel: [w394 w401] -> w388
              tunnel: [w393 w400] -> w387
              tunnel: w386 -> [_ w399]
              tunnel: w385 -> [_ w398]
              tunnel: w381 -> [_ w395]
              frame False {
              }
              frame True {
                n138 = Add(x=w398, y=w399) -> (x+y=w397:dbl)
                n139 = global read "RIO and DAC defaults global.vi" "TTL pulse duration (ms)"() -> (w396:dbl)
                n140 = case shown="2" w395 {
                  tunnel: w405 -> [w414 w420 w426]
                  tunnel: [w409 w421 w424] -> w400
                  tunnel: w396 -> [w410 w418 w425]
                  tunnel: w397 -> [w408 w417 w427]
                  frame 0, Default {
                    w411 = TRUE ("Do this?")
                    n141 = global read "RIO and DAC defaults global.vi" "Port"() -> (w407:i32)
                    n142 = Add(x=w408, y=w410) -> (x+y=w413:dbl)
                    n143 = global read "RIO and DAC defaults global.vi" "Line"() -> (w406:i32)
                    n144 = call "TTL high.vi"("Line"=w406, "Port"=w407, "Do this?"=w411, "Input"=w414, "Absolute start time (ms)"=w408) -> ("Output"=w412:i64[][])
                    n145 = call "TTL low.vi"("Line"=w406, "Port"=w407, "Do this?"=w411, "Input"=w412, "Absolute start time (ms)"=w413) -> ("Output"=w409:i64[][])
                  }
                  frame 1 {
                    w419 = TRUE ("Do this?")
                    n146 = global read "RIO and DAC defaults global.vi" "Port 2"() -> (w416:i32)
                    n147 = Add(x=w417, y=w418) -> (x+y=w422:dbl)
                    n148 = global read "RIO and DAC defaults global.vi" "Line 2"() -> (w415:i32)
                    n149 = call "TTL high.vi"("Line"=w415, "Port"=w416, "Do this?"=w419, "Input"=w420, "Absolute start time (ms)"=w417) -> ("Output"=w423:i64[][])
                    n150 = call "TTL low.vi"("Line"=w415, "Port"=w416, "Do this?"=w419, "Input"=w423, "Absolute start time (ms)"=w422) -> ("Output"=w421:i64[][])
                  }
                  frame 2 {
                    w430 = TRUE ("Do this?")
                    n151 = global read "RIO and DAC defaults global.vi" "Port 3"() -> (w429:i32)
                    n152 = Add(x=w427, y=w425) -> (x+y=w431:dbl)
                    n153 = global read "RIO and DAC defaults global.vi" "Line 3"() -> (w428:i32)
                    n154 = call "TTL high.vi"("Line"=w428, "Port"=w429, "Do this?"=w430, "Input"=w426, "Absolute start time (ms)"=w427) -> ("Output"=w432:i64[][])
                    n155 = call "TTL low.vi"("Line"=w428, "Port"=w429, "Do this?"=w430, "Input"=w432, "Absolute start time (ms)"=w431) -> ("Output"=w424:i64[][])
                  }
                }
                n156 = call "Static DAC cluster generator.vi"("time entry"=w397, "voltage entry"=w403, "DAQ channel\n number"=w402, "Input Array"=w404) -> ("Output Array"=w401:T1)
              }
            }
          }
          "Static input 2" <- w269
          n157 = for {
            tunnel: w270 -> [w315] mode=indexing
            shift-right: [w313] -> w268
            shift-left: w269 -> [w314]
            shift-right: [w310] -> w265
            shift-left: w266 -> [w311]
            tunnel: w261 -> [w309]
            n158 = Unbundle By Name(w315) -> ("Write Ramp?"=w316:bool, "DAC Channel"=w312:i16)
            n159 = for {
              tunnel: w316 -> [w322]
              tunnel: w315 -> [w327]
              tunnel: w314 -> [w326] mode=indexing
              tunnel: [w325] -> w313 mode=indexing
              tunnel: w312 -> [w321]
              shift-right: [w318] -> w310
              shift-left: w311 -> [w319]
              tunnel: w309 -> [w317]
              i -> [w324]
              # "This loops through the DAC channels"
              n160 = Equal?(x=w321, y=w324) -> (x = y?=w323:bool)
              n161 = And(x=w322, y=w323) -> (x .and. y?=w320:bool)
              n162 = case shown="True" w320 {
                tunnel: w327 -> [_ w346]
                tunnel: w326 -> [w329 w345]
                tunnel: [w329 w339] -> w325
                tunnel: w319 -> [w328 w336]
                tunnel: [w328 w335] -> w318
                tunnel: w321 -> [_ w334]
                tunnel: w317 -> [_ w332]
                frame False {
                }
                frame True {
                  # "This calculates times and voltages for the linear DAC ramps"
                  n163 = Unbundle By Name(w345) -> ("Times"=w344:dbl[], "Voltages"=w343:dbl[])
                  n164 = call "Linear ramp.vi"("Input"=w346) -> ("Time Array"=w333:dbl[], "Volt Array"=w342:dbl[])
                  n165 = Add(x=w333, y=w332) -> (x+y=w331:dbl[])
                  n166 = global read "RIO and DAC defaults global.vi" "TTL pulse duration (ms)"() -> (w330:dbl)
                  n167 = for {
                    tunnel: w330 -> [w353]
                    tunnel: w331 -> [w352] mode=indexing
                    shift-right: [w350] -> w335
                    shift-left: w336 -> [w351]
                    tunnel: w334 -> [w347]
                    n168 = Quotient & Remainder(x=w347, y=8) -> (floor(x/y)=w348:i32)  [unwired: 1 out]
                    n169 = case shown="2" w348 {
                      tunnel: [w358 w369 w372] -> w350
                      tunnel: w353 -> [w359 w367 w373]
                      tunnel: w352 -> [w357 w366 w375]
                      tunnel: w351 -> [w356 w365 w374]
                      frame 0, Default {
                        w360 = TRUE ("Do this?")
                        n170 = global read "RIO and DAC defaults global.vi" "Port"() -> (w355:i32)
                        n171 = Add(x=w357, y=w359) -> (x+y=w362:dbl)
                        n172 = global read "RIO and DAC defaults global.vi" "Line"() -> (w354:i32)
                        n173 = call "TTL high.vi"("Line"=w354, "Port"=w355, "Do this?"=w360, "Input"=w356, "Absolute start time (ms)"=w357) -> ("Output"=w361:i64[][])
                        n174 = call "TTL low.vi"("Line"=w354, "Port"=w355, "Do this?"=w360, "Input"=w361, "Absolute start time (ms)"=w362) -> ("Output"=w358:i64[][])
                      }
                      frame 1 {
                        w368 = TRUE ("Do this?")
                        n175 = global read "RIO and DAC defaults global.vi" "Port 2"() -> (w364:i32)
                        n176 = Add(x=w366, y=w367) -> (x+y=w370:dbl)
                        n177 = global read "RIO and DAC defaults global.vi" "Line 2"() -> (w363:i32)
                        n178 = call "TTL high.vi"("Line"=w363, "Port"=w364, "Do this?"=w368, "Input"=w365, "Absolute start time (ms)"=w366) -> ("Output"=w371:i64[][])
                        n179 = call "TTL low.vi"("Line"=w363, "Port"=w364, "Do this?"=w368, "Input"=w371, "Absolute start time (ms)"=w370) -> ("Output"=w369:i64[][])
                      }
                      frame 2 {
                        w378 = TRUE ("Do this?")
                        n180 = global read "RIO and DAC defaults global.vi" "Port 3"() -> (w377:i32)
                        n181 = Add(x=w375, y=w373) -> (x+y=w379:dbl)
                        n182 = global read "RIO and DAC defaults global.vi" "Line 3"() -> (w376:i32)
                        n183 = call "TTL high.vi"("Line"=w376, "Port"=w377, "Do this?"=w378, "Input"=w374, "Absolute start time (ms)"=w375) -> ("Output"=w380:i64[][])
                        n184 = call "TTL low.vi"("Line"=w376, "Port"=w377, "Do this?"=w378, "Input"=w380, "Absolute start time (ms)"=w379) -> ("Output"=w372:i64[][])
                      }
                    }
                  }
                  n185 = Insert Into Array(array=w343, new element=w342) -> (w338:dbl[])  [unwired: 1 in]
                  n186 = Insert Into Array(array=w344, new element=w331) -> (w340:dbl[])  [unwired: 1 in]
                  n187 = Array Size(array=w338) -> (size(s)=w337:i32)
                  n188 = Bundle By Name(cluster=w345, "Times"=w340, "Voltages"=w338, "Enable Ch"=TRUE, "Hinge Points"=w337) -> (w339:T16)
                }
              }
            }
          }
          "Array" <- w271
        }
      }
      "Output" <- w185
      "Static output" <- w187
      "GPIB Output" <- w180
    }
  }
